vi "zmq_setsocketopt.vi"(4 "error in":errorcluster, 5 "value":variant, 6 "option":T1=enum."ZMQ_SWAP", 7 "socket in":refnum<class "zmq_socket.lvclass">) -> (0 "error out":errorcluster, 3 "socket out":refnum<class "zmq_socket.lvclass">)   [LabVIEW 2010, in "zeromq.lvlib" / "zmq_socket.lvclass"]
doc: "Sets the specified <b>option</b> to the given <b>value</b>. The type of data connected to value must match that expected by the option (see the API documentation).\n\nNote that LabVIEW strings are used for \"raw\" data.\n\nDetailed API documentation: http://api.zeromq.org/3-2:zmq-setsockopt"
uses:
  zmq_socket.lvclass
  socket_options.ctl
  zmq_socket.lvclass/zmq_socket.ctl
  zeromq.lvlib
panel:
  out "option code":i32
  # "ØMQ"
  # "labview"
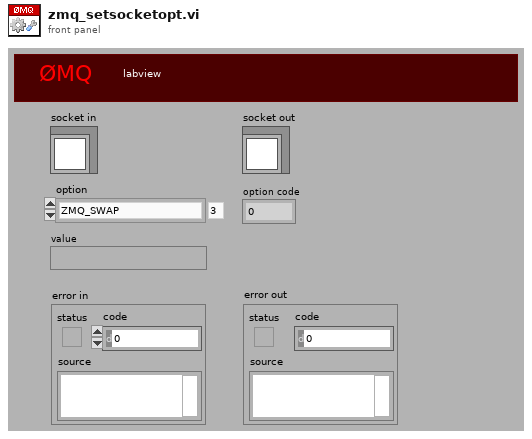
[diagram p1: front panel]
types:
  T1 = typedef "zeromq.lvlib/socket_options.ctl" = enum8{"NONE", "ZMQ_HWM", "<2>", "ZMQ_SWAP", "ZMQ_AFFINITY", "ZMQ_IDENTITY", "ZMQ_SUBSCRIBE", "ZMQ_UNSUBSCRIBE", "ZMQ_RATE", "ZMQ_RECOVERY_IVL", "ZMQ_MCAST_LOOP", "ZMQ_SNDBUF", "ZMQ_RCVBUF", "ZMQ_RCVMORE", "ZMQ_FD", "ZMQ_EVENTS", "ZMQ_TYPE", "ZMQ_LINGER", "ZMQ_RECONNECT_IVL", "ZMQ_BACKLOG", "ZMQ_RECOVERY_IVL_MSEC", "ZMQ_RECONNECT_IVL_MAX", "ZMQ_MAXMSGSIZE", "ZMQ_SNDHWM", "ZMQ_RCVHWM", "ZMQ_MULTICAST_HOPS", "<26>", "ZMQ_RCVTIMEO", "ZMQ_SNDTIMEO", "<29>", "<30>", "ZMQ_IPV4ONLY", "ZMQ_LAST_ENDPOINT", "ZMQ_ROUTER_MANDATORY", "ZMQ_TCP_KEEPALIVE", "ZMQ_TCP_KEEPALIVE_CNT", "ZMQ_TCP_KEEPALIVE_IDLE", "ZMQ_TCP_KEEPALIVE_INTVL", "ZMQ_TCP_ACCEPT_FILTER", "ZMQ_DELAY_ATTACH_ON_CONNECT", "ZMQ_XPUB_VERBOSE"}
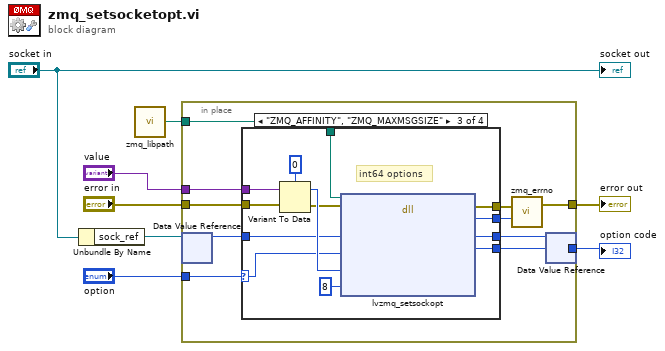
[diagram p0: block diagram]
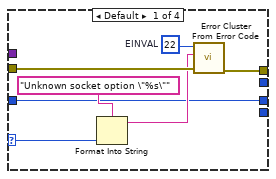
[diagram p2: hidden frame]
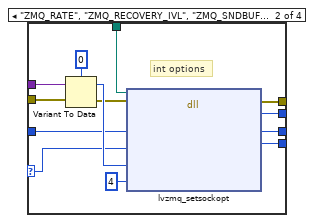
[diagram p3: hidden frame]
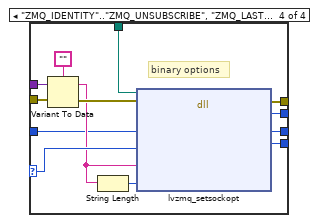
[diagram p4: hidden frame]
diagram:
  n1 = Unbundle By Name("socket in") -> ("sock_ref"=w2:refnum<data-value>)
  n2 = call "zmq_libpath.vi"() -> ("path"=w1:path)
  n3 = in-place {
    in-place-border: [w16] -> w8
    in-place-border: "value" -> [w15]
    in-place-border: "error in" -> [w14]
    in-place-border: "option" -> [w13]
    in-place-border: [w12] -> w4
    in-place-border: w1 -> [w9]
    n4 = in-place-dvr #1(w2) -> (w11:u64)  [unwired: 1 out]
    n5 = case shown="\"ZMQ_AFFINITY\", \"ZMQ_MAXMSGSIZE\"" w13 {
      selector: w13 -> [w22 w31 w44 w58]
      tunnel: [w25 w38 w51 w64] -> w18
      tunnel: [_ w37 w50 w63] -> w17
      tunnel: w15 -> [_ w36 w49 w62]
      tunnel: w14 -> [w23 w33 w46 w60]
      tunnel: [_ w29 w42 w55] -> w12
      tunnel: w11 -> [w19 w28 w41 w53]
      tunnel: [w19 w27 w40 w54] -> w10
      tunnel: w9 -> [_ w26 w39 w52]
      frame Default {
        w24 = 22  # EINVAL
        n6 = Format Into String(format string="Unknown socket option \"%s\"", w22) -> (resulting string=w20:string)  [unwired: 2 in, 1 out]
        n7 = call <vilib>:"Error Cluster From Error Code.vi"("error in (no error)"=w23, "error message (\"\")"=w20, "error code (0)"=w24) -> ("error out"=w25:errorcluster)  [unwired: 6 in]
      }
      frame "ZMQ_RATE", "ZMQ_RECOVERY_IVL", "ZMQ_SNDBUF".."ZMQ_RECONNECT_IVL_MAX", "ZMQ_SNDHWM".."ZMQ_MULTICAST_HOPS", "ZMQ_RCVTIMEO", "ZMQ_SNDTIMEO", "ZMQ_IPV4ONLY", "ZMQ_ROUTER_MANDATORY".."ZMQ_XPUB_VERBOSE" {
        # "int options"
        n8 = Variant To Data(error in=w33, Variant=w36, type=0) -> (error out=w32:errorcluster, data=w35:i32)
        n9 = dll-call lib="?" fn="lvzmq_setsockopt"(path in=w26, error in=w32, "socket"=w28, "option"=w31, "data"=w35, "len"=u32 4) -> (error out=w38:errorcluster, "return type"=w37:i32, "socket"=w27:u64, "option"=w29:i32)  [unwired: 3 in, 1 out]
      }
      frame "ZMQ_AFFINITY", "ZMQ_MAXMSGSIZE" {
        # "int64 options"
        n10 = Variant To Data(error in=w46, Variant=w49, type=i64 0) -> (error out=w45:errorcluster, data=w48:i64)
        n11 = dll-call lib="?" fn="lvzmq_setsockopt"(path in=w39, error in=w45, "socket"=w41, "option"=w44, "data"=w48, "len"=u32 8) -> (error out=w51:errorcluster, "return type"=w50:i32, "socket"=w40:u64, "option"=w42:i32)  [unwired: 3 in, 1 out]
      }
      frame "ZMQ_IDENTITY".."ZMQ_UNSUBSCRIBE", "ZMQ_LAST_ENDPOINT" {
        # "binary options"
        n12 = Variant To Data(error in=w60, Variant=w62, type="") -> (error out=w59:errorcluster, data=w56:string)
        n13 = String Length(string=w56) -> (length=w57:i32)
        n14 = dll-call lib="?" fn="lvzmq_setsockopt"(path in=w52, error in=w59, "socket"=w53, "option"=w58, "data"=w56, "len"=w57) -> (error out=w64:errorcluster, "return type"=w63:i32, "socket"=w54:u64, "option"=w55:i32)  [unwired: 3 in, 1 out]
      }
    }
    n15 = call "zmq_errno.vi"("retval"=w17, "error in"=w18) -> ("error out"=w16:errorcluster)  [unwired: 1 out]
    n16 = in-place-dvr #1(w10) -> ()  [unwired: 2 out]
  }
  "error out" <- w8
  "option code" <- w4
  "socket out" <- "socket in"
